vi "zamknijI2C.vi"(5 "Close I2C Master?":bool, 7 "I2C Channel (0)":u8, 8 "Error In":errorcluster, 10 "I2C Slave Address (0)":u8, 11 "LINX Resource":T1) -> (0 "Error Out":errorcluster, 3 "LINX Resource":T1)   [LabVIEW 2014]
doc: "Close the MMA8452 and optionally close the I2C master."
uses:
  <vilib>/MakerHub/LINX/LMH-LINX.lvlib
  czytajI2CVIs/usrednijVIs/AkcjaUsredniania.ctl
  <vilib>/MakerHub/LINX/Private/Type Defs/Platform.ctl
  <vilib>/MakerHub/LINX/Private/Type Defs/Interface.ctl
  <vilib>/MakerHub/LINX/Private/Device/Type Defs/TCP Config.ctl
  <vilib>/MakerHub/LINX/Private/Device/Device.lvlib
  <vilib>/MakerHub/LINX/Private/Device/Type Defs/Channels.ctl
  <vilib>/MakerHub/LINX/Private/Device/Type Defs/LINX Device Config.ctl
  <vilib>/MakerHub/LINX/Private/Type Defs/LINX Ref.ctl
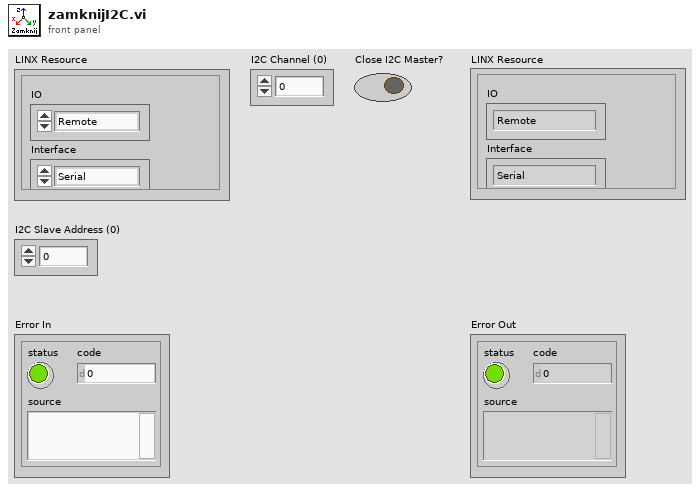
[diagram p1: front panel]
types:
  T1 = typedef "LMH-LINX.lvlib/LINX Ref.ctl" = cluster{"IO":T2, "Interface":T3, "LINX Device Config":T4}
  T2 = typedef "LMH-LINX.lvlib/Platform.ctl" = enum16{"Remote", "Local"}
  T3 = typedef "LMH-LINX.lvlib/Interface.ctl" = enum16{"Serial", "TCP"}
  T4 = typedef "LMH-LINX.lvlib/Device.lvlib/LINX Device Config.ctl" = cluster{"Interface":T3, "COM Port":refnum<visa-resource-name>, "TCP Configuration":T5, "Device Family":u8, "Device ID":u8, "Device Name":string, "TCP Ref":refnum<k5>, "Channels":T6}
  T5 = typedef "LMH-LINX.lvlib/Device.lvlib/TCP Config.ctl" = cluster{"IP Address":string, "Port":u16}
  T6 = typedef "LMH-LINX.lvlib/Channels.ctl" = cluster{"DI":u8[], "DO":u8[], "AI":u8[], "AO":u8[], "PWM":u8[], "QE":u8[], "UART":u8[], "I2C 2":u8[], "SPI":u8[], "CAN":u8[], "Servo":u8[], "AI Ref (V)":dbl, "AI Resolution (Bits)":u8, "AO Ref (V)":dbl, "AO Resolution (Bits)":u8}
  T7 = typedef "AkcjaUsredniania.ctl" = enum16{"Init", "DodajWartość", "WypełnijKolejkę", "Koniec"}
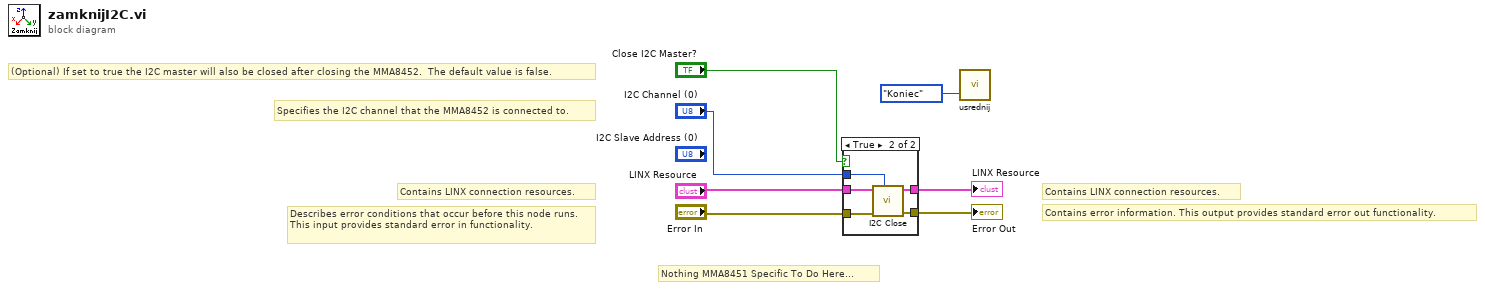
[diagram p0: block diagram]
diagram:
  # "Specifies the I2C channel that the MMA8452 is connected to."
  # "(Optional) If set to true the I2C master will also be closed after closing the MMA8452.  The default value is false."
  # "Contains LINX connection resources."
  # "Describes error conditions that occur before this node runs. This input provides standard error in functionality."
  # "Contains LINX connection resources."
  # "Contains error information. This output provides standard error out functionality."
  # "Nothing MMA8451 Specific To Do Here..."
  n1 = case shown="True" "Close I2C Master?" {
    tunnel: [w9 w14] -> w7
    tunnel: [w8 w13] -> w6
    tunnel: "LINX Resource" -> [w9 w12]
    tunnel: "Error In" -> [w8 w11]
    tunnel: "I2C Channel (0)" -> [_ w10]
    frame False {
    }
    frame True {
      n2 = call <vilib>:"I2C Close.vi"("I2C Channel (0)"=w10, "Error In"=w11, "LINX Resource"=w12) -> ("Error Out"=w13:errorcluster, "LINX Resource"=w14:T1)  [unwired: 7 in]
    }
  }
  "Error Out" <- w6
  "LINX Resource" <- w7
  n3 = call "usrednij.vi"("AkcjaUsredniania"=AkcjaUsredniania."Koniec") -> ()  [unwired: 1 in, 2 out]
